vi "hpanel_write_control_references.vi"(8 "error in (no error)":errorcluster, 10 "references":T1, 11 "hydraharp_panel in":refnum<class "hydraharp_panel.lvclass">) -> (0 "error out":errorcluster, 3 "hydraharp_panel out":refnum<class "hydraharp_panel.lvclass">)   [LabVIEW 2015, in "hydraharp_panel.lvclass"]
uses:
  hydraharp_panel.lvclass
  hpanel_control_references.ctl
  hydraharp_panel.lvclass/hydraharp_panel.ctl
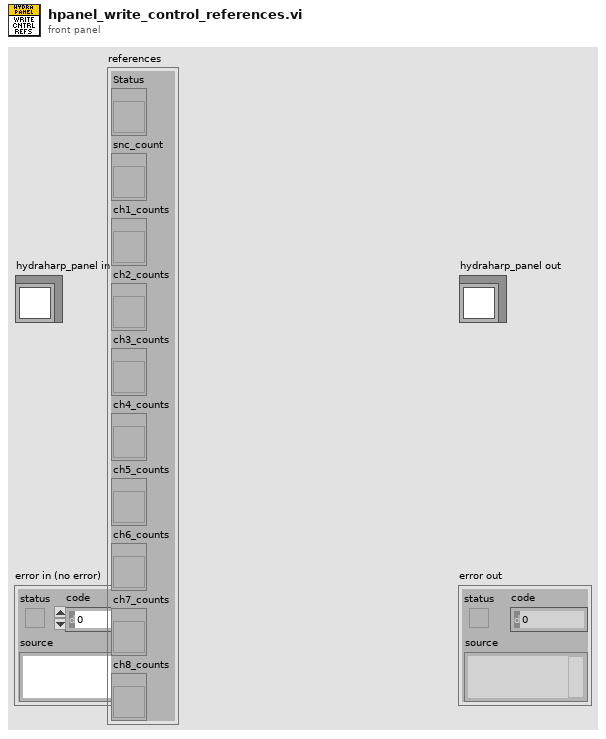
[diagram p1: front panel]
types:
  T1 = typedef "hpanel_control_references.ctl" = cluster{"Status":refnum<vi>, "snc_count":refnum<vi>, "ch1_counts":refnum<vi>, "ch2_counts":refnum<vi>, "ch3_counts":refnum<vi>, "ch4_counts":refnum<vi>, "ch5_counts":refnum<vi>, "ch6_counts":refnum<vi>, "ch7_counts":refnum<vi>, "ch8_counts":refnum<vi>}
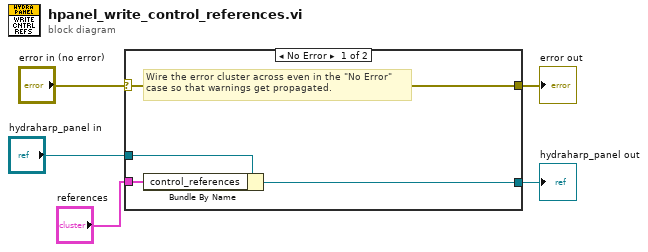
[diagram p0: block diagram]
diagram:
  n1 = case shown="No Error" "error in (no error)" {
    selector: "error in (no error)" -> [w9 w11]
    tunnel: [w9 w11] -> w4
    tunnel: [w7 w10] -> w2
    tunnel: "hydraharp_panel in" -> [w8 w10]
    tunnel: "references" -> [w6 _]
    frame No Error {
      # "Wire the error cluster across even in the \"No Error\"\ncase so that warnings get propagated."
      n2 = Bundle By Name(cluster=w8, "control_references"=w6) -> (w7:refnum<class "hydraharp_panel.lvclass">)
    }
    frame Error {
    }
  }
  "error out" <- w4
  "hydraharp_panel out" <- w2
